vi "主程序.vi"() -> ()   [LabVIEW 2018]
uses:
  <vilib>/vision/NI_Vision_Development_Module.lvlib
panel:
  out "项目路径":path
  out "分析图":cluster{"x0":sgl, "dx":sgl, "Pixels Line":sgl[]}(graph)
  in  "选项卡":enum32{"图像处理", "灰度处理"}(tab)
  in  "打开图像":bool
  in  "转换灰度图":bool
  in  "裁剪ROI":bool
  in  "图像变换":bool
  in  "线灰度曲线":bool
  in  "直方图":bool
  in  "结构相似性":bool
  in  "灰度变换":bool
  out "图像":T1(plugin-control)
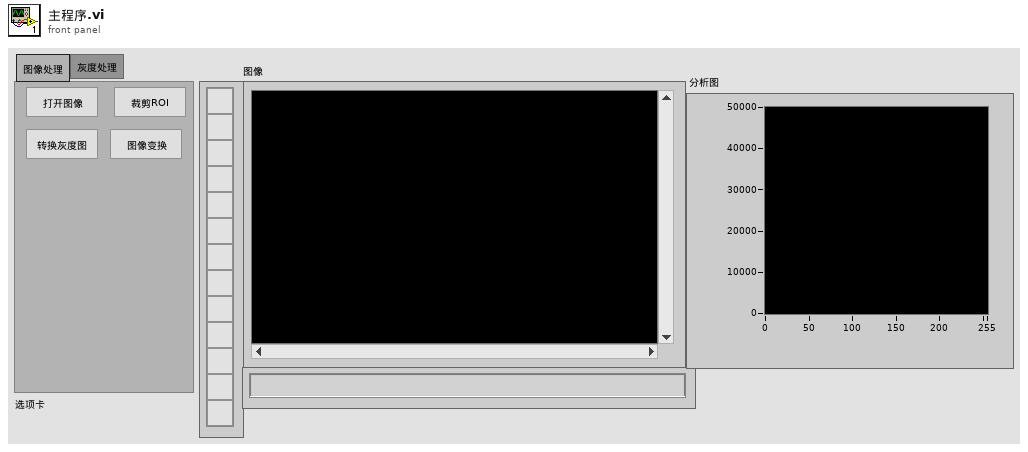
[diagram p1: front panel]
types:
  T1 = typedef "IMAQ Image.ctl" = refnum<image>
  T2 = cluster{"Global Rectangle":i32[], "Contours":cluster{"Contour Type":u32, "ROI Type":u32, "Points":i32[]}[]}
  T3 = typedef "Image Type" = u32
  T4 = cluster{"移动x":dbl, "移动y":dbl, "旋转角度":dbl, "是否镜像":bool, "镜像方法":u32}
  T5 = cluster{"Starting Value":sgl, "Incremental Value":sgl, "Histogram":u32[]}
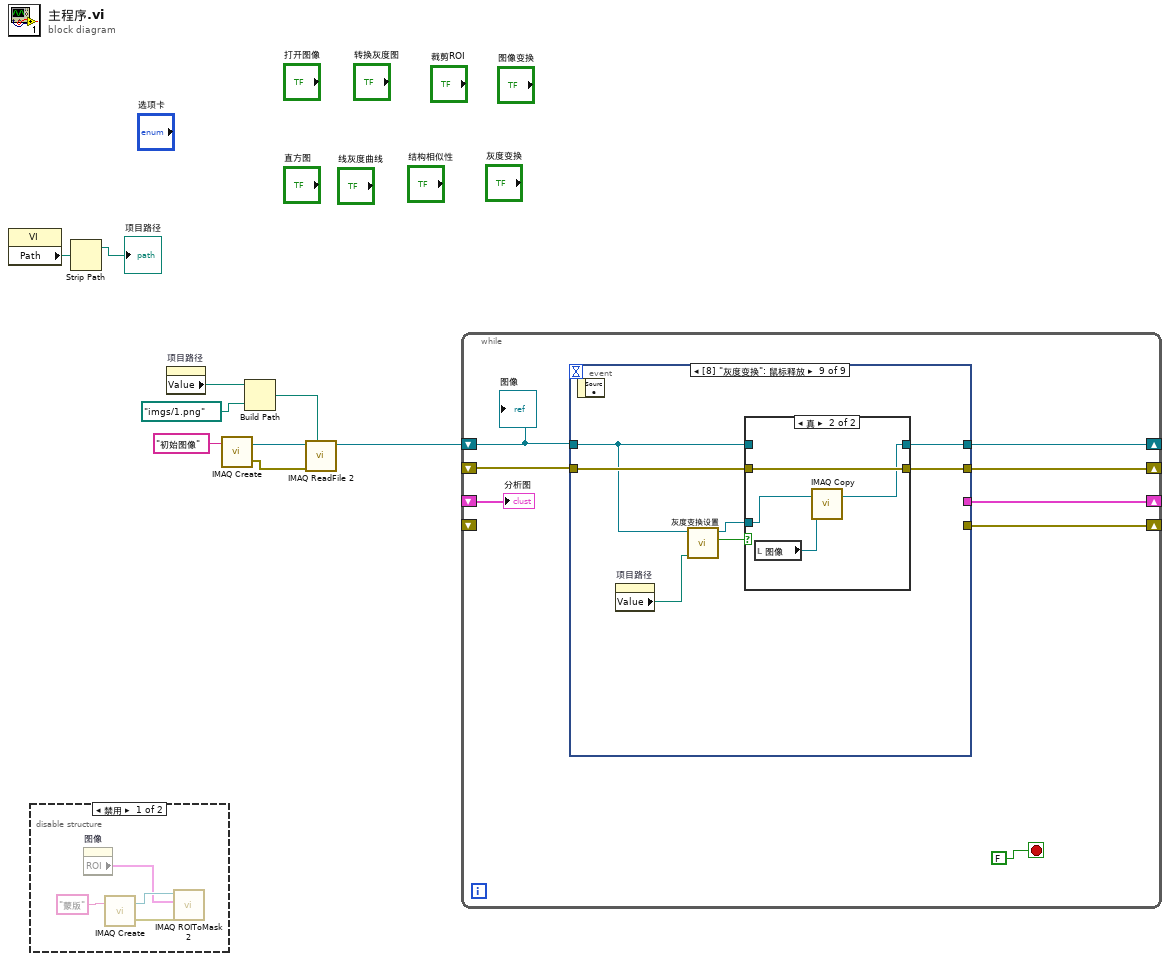
[diagram p0: block diagram]
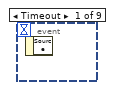
[diagram p3: hidden frame]
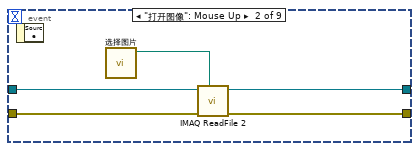
[diagram p4: hidden frame]
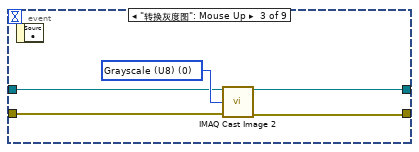
[diagram p5: hidden frame]
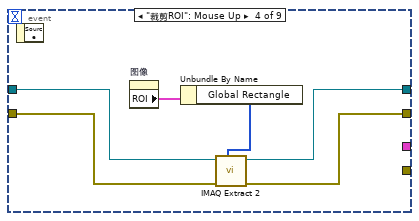
[diagram p6: hidden frame]
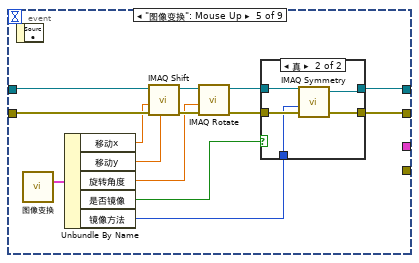
[diagram p7: hidden frame]
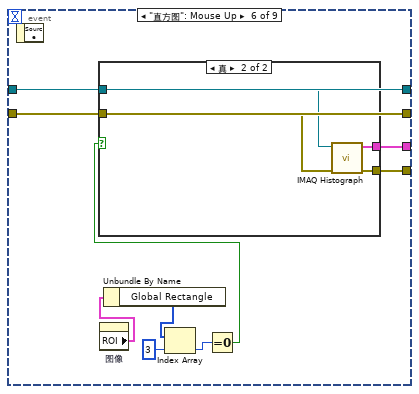
[diagram p9: hidden frame]
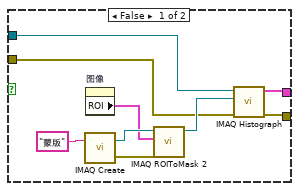
[diagram p10: hidden frame]
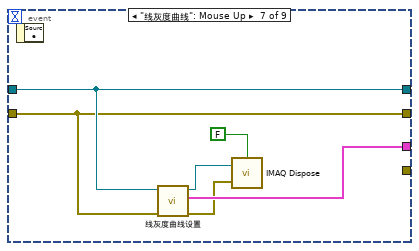
[diagram p11: hidden frame]
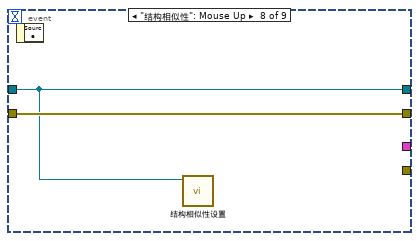
[diagram p12: hidden frame]
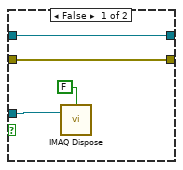
[diagram p13: hidden frame]
diagram:
  n1 = property class="VI"() -> ("Path"=w5:path)  [unwired: 2 in, 2 out]
  n2 = disable-structure shown="禁用" {
    frame Disabled {
      n3 = property on="图像" class="ImageControl"() -> ("ROI"=w10:T2)  [unwired: 2 in, 2 out]
      n4 = call "IMAQ Create"("Image Name"="蒙版") -> ("New Image"=w12:T1, "error out"=w13:errorcluster)  [unwired: 4 in]
      n5 = call "IMAQ ROIToMask 2"("error in (no error)"=w13, "ROI Descriptor"=w10, "Image"=w12) -> ()  [unwired: 6 in, 3 out]
    }
    frame Enabled {
    }
  }
  n6 = Strip Path(path=w5) -> (stripped path=→"项目路径":path)  [unwired: 1 out]
  n7 = property on="项目路径" class="Path"() -> ("Value"=w3:path)  [unwired: 2 in, 2 out]
  n8 = call "IMAQ Create"("Image Name"="初始图像") -> ("New Image"=w7:T1, "error out"=w8:errorcluster)  [unwired: 4 in]
  n9 = Build Path(base path=w3, name or relative path=path "imgs/1.png" ("路径")) -> (appended path=w1:path)
  n10 = call "IMAQ ReadFile 2"("File Path"=w1, "error in (no error)"=w8, "Image"=w7) -> ("Image Out"=w6:T1)  [unwired: 4 in, 4 out]
  n11 = while {
    shift-right: [w20] -> _
    shift-left: w6 -> [w19]
    shift-right: [w21] -> _
    shift-left: _ -> [w18]
    shift-right: [w17] -> _
    shift-left: _ -> [w15]
    shift-right: [w16] -> _
    shift-left: _ -> [_]
    stop <- FALSE stop-if-true
    n12 = event shown="[8] \"灰度变换\": 鼠标释放" {
      selector: _ -> [_ _ _ _ _ _ _ _ _]
      dyn-events: _ -> [_ _ _ _ _ _ _ _ _]
      timeout: _ -> [_ _ _ _ _ _ _ _ _]
      tunnel: [_ w26 w29 w36 w40 w67 w86 w87 w94] -> w20
      tunnel: [_ w25 w28 w35 w39 w66 w85 w88 w92] -> w21
      tunnel: w18 -> [_ w24 w30 w34 w51 w66 w85 w88 w93]
      tunnel: w19 -> [_ w23 w27 w33 w48 w67 w86 w87 w90]
      tunnel: [_ _ _ _ _ w65 w84 _ _] -> w17
      tunnel: [_ _ _ _ _ w64 _ _ _] -> w16
      event Timeout {
        n13 = event-data() -> ()  [unwired: 1 in, 1 out]
      }
      event "打开图像": Mouse Up {
        n14 = event-data() -> ()  [unwired: 1 in, 1 out]
        n15 = call "选择图片.vi"() -> ("图像路径 2"=w22:path)  [unwired: 11 in]
        n16 = call "IMAQ ReadFile 2"("File Path"=w22, "error in (no error)"=w24, "Image"=w23) -> ("error out"=w25:errorcluster, "Image Out"=w26:T1)  [unwired: 4 in, 3 out]
      }
      event "转换灰度图": Mouse Up {
        w31 = T3 0 items=["Grayscale (U8)", "Grayscale (I16)", "Grayscale (SGL)", "Complex (CSG)", "RGB (U32)", "HSL (U32)", "RGB (U64)", "Grayscale (U16)"] ("Image Type")
        n17 = event-data() -> ()  [unwired: 1 in, 1 out]
        n18 = call "IMAQ Cast Image 2"("Image Src"=w27, "Image Type"=w31, "error in (no error)"=w30) -> ("Image Dst Out"=w29:T1, "error out"=w28:errorcluster)  [unwired: 11 in]
      }
      event "裁剪ROI": Mouse Up {
        n19 = event-data() -> ()  [unwired: 1 in, 1 out]
        n20 = property on="图像" class="ImageControl"() -> ("ROI"=w32:T2)  [unwired: 2 in, 2 out]
        n21 = Unbundle By Name(w32) -> ("Global Rectangle"=w37:i32[])
        n22 = call "IMAQ Extract 2"("Optional Rectangle"=w37, "error in (no error)"=w34, "Image Src"=w33) -> ("error out"=w35:errorcluster, "Image Dst Out"=w36:T1)  [unwired: 7 in]
      }
      event "图像变换": Mouse Up {
        n23 = event-data() -> ()  [unwired: 1 in, 1 out]
        n24 = call "图像变换.vi"() -> ("簇"=w47:T4)  [unwired: 11 in]
        n25 = Unbundle By Name(w47) -> ("移动x"=w46:dbl, "移动y"=w45:dbl, "旋转角度"=w44:dbl, "是否镜像"=w43:bool, "镜像方法"=w38:u32)
        n26 = call "IMAQ Shift"("YOffset"=w45, "error in (no error)"=w51, "XOffset"=w46, "Image Src"=w48) -> ("error out"=w50:errorcluster, "Image Dst Out"=w49:T1)  [unwired: 6 in]
        n27 = call "IMAQ Rotate"("error in (no error)"=w50, "Angle (degrees)"=w44, "Image Src"=w49) -> ("error out"=w41:errorcluster, "Image Dst Out"=w42:T1)  [unwired: 7 in]
        n28 = case shown="真" w43 {
          tunnel: w42 -> [w53 w58]
          tunnel: w41 -> [w52 w57]
          tunnel: [w53 w56] -> w40
          tunnel: [w52 w55] -> w39
          tunnel: w38 -> [_ w54]
          frame False {
          }
          frame True {
            n29 = call "IMAQ Symmetry"("error in (no error)"=w57, "Type of Symmetry"=w54, "Image Src"=w58) -> ("error out"=w55:errorcluster, "Image Dst Out"=w56:T1)  [unwired: 2 in]
          }
        }
      }
      event "直方图": Mouse Up {
        n30 = event-data() -> ()  [unwired: 1 in, 1 out]
        n31 = property on="图像" class="ImageControl"() -> ("ROI"=w60:T2)  [unwired: 2 in, 2 out]
        n32 = Unbundle By Name(w60) -> ("Global Rectangle"=w62:i32[])
        n33 = Index Array(array=w62, index=3 ("索引")) -> (element=w61:i32)
        n34 = Equal To 0?(x=w61) -> (x = 0?=w59:bool)
        n35 = case shown="真" w59 {
          tunnel: w67 -> [w69 w80]
          tunnel: w66 -> [w68 w79]
          tunnel: [w71 w78] -> w65
          tunnel: [w70 w77] -> w64
          frame False {
            n36 = call "IMAQ Create"("Image Name"="蒙版") -> ("New Image"=w75:T1, "error out"=w74:errorcluster)  [unwired: 4 in]
            n37 = property on="图像" class="ImageControl"() -> ("ROI"=w72:T2)  [unwired: 2 in, 2 out]
            n38 = call "IMAQ ROIToMask 2"("error in (no error)"=w74, "ROI Descriptor"=w72, "Image"=w75) -> ("Image Out"=w73:T1)  [unwired: 6 in, 2 out]
            n39 = call "IMAQ Histograph"("error in (no error)"=w68, "Image Mask"=w73, "Image"=w69) -> ("error out"=w70:errorcluster, "Histogram Graph"=w71:T5)  [unwired: 5 in, 2 out]
          }
          frame True {
            n40 = call "IMAQ Histograph"("error in (no error)"=w79, "Image"=w80) -> ("error out"=w77:errorcluster, "Histogram Graph"=w78:T5)  [unwired: 6 in, 2 out]
          }
        }
      }
      event "线灰度曲线": Mouse Up {
        n41 = event-data() -> ()  [unwired: 1 in, 1 out]
        n42 = call "线灰度曲线设置.vi"("error in (no error)"=w85, "Image Src"=w86) -> ("error out"=w81:errorcluster, "分析图"=w84:cluster{"x0":sgl, "dx":sgl, "Pixels Line":sgl[]}, "图像"=w82:T1)  [unwired: 7 in]
        n43 = call "IMAQ Dispose"("All Images? (No)"=FALSE, "Image"=w82, "error in (no error)"=w81) -> ()  [unwired: 3 in, 1 out]
      }
      event "结构相似性": Mouse Up {
        n44 = event-data() -> ()  [unwired: 1 in, 1 out]
        n45 = call "结构相似性设置.vi"("图像输入"=w87) -> ()  [unwired: 9 in, 2 out]
      }
      event "灰度变换": Mouse Up {
        n46 = event-data() -> ()  [unwired: 1 in, 1 out]
        n47 = property on="项目路径" class="Path"() -> ("Value"=w89:path)  [unwired: 2 in, 2 out]
        n48 = call "灰度变换设置.vi"("项目路径"=w89, "图像输入"=w90) -> ("是否应用"=w95:bool, "图像"=w91:T1)  [unwired: 8 in]
        n49 = case shown="真" w95 {
          tunnel: [w99 w100] -> w94
          tunnel: w90 -> [w99 _]
          tunnel: [w98 w103] -> w92
          tunnel: w93 -> [w98 w103]
          tunnel: w91 -> [w96 w101]
          frame False {
            n50 = call "IMAQ Dispose"("All Images? (No)"=FALSE, "Image"=w96) -> ()  [unwired: 4 in, 1 out]
          }
          frame True {
            n51 = local read "图像"() -> (w102:T1)
            n52 = call "IMAQ Copy"("Image Dst"=w102, "Image Src"=w101) -> ("Image Dst Out"=w100:T1)  [unwired: 4 in, 1 out]
          }
        }
      }
    }
    "图像" <- w19
    "分析图" <- w15
  }
